vi "Set value notation.vi"(8 "error in":errorcluster, 10 "Calibration mode (disable)":u16(ring) items=["Scientific with legends", "Scientific with no legends", "Engeneering with legends", "Engeneering without legends"], 11 "VISA resource name":refnum<visa-resource-name>) -> (0 "error out":errorcluster, 3 "VISA resource name out":refnum<visa-resource-name>)   [LabVIEW 2012, in "Datron D4xxx.lvlib"]
doc: "This VI sets instrument number format."
uses:
  Datron D4xxx.lvlib
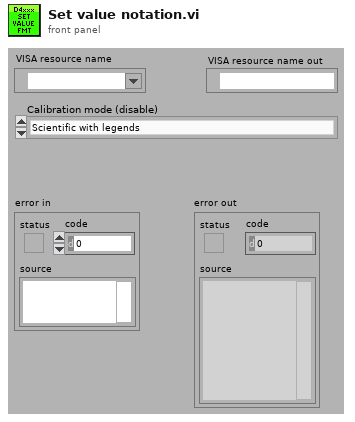
[diagram p1: front panel]
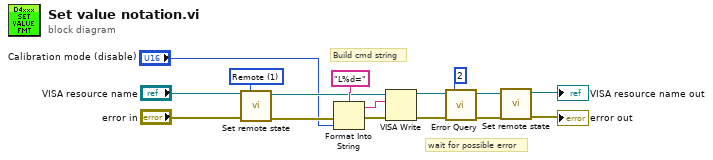
[diagram p0: block diagram]
diagram:
  w3 = u16 1 items=["Local", "Remote", "Default"] ("Remote state")
  # "Build cmd string"
  # "wait for possible error"
  n1 = call "Set remote state.vi"("error in"="error in", "Remote state"=w3, "VISA resource name"="VISA resource name") -> ("error out"=w6:errorcluster, "VISA resource name out"=w4:refnum<visa-resource-name>)  [unwired: 7 in]
  n2 = Format Into String(format string="L%d=", error in=w6, "Calibration mode (disable)") -> (resulting string=w16:string, error out=w15:errorcluster)  [unwired: 1 in]
  n3 = VISA Write(VISA resource name=w4, write buffer=w16, error in (no error)=w15) -> (VISA resource name out=w8:refnum<visa-resource-name>, error out=w9:errorcluster)  [unwired: 1 out]
  n4 = call "Error Query.vi"("error in (no error)"=w9, "Check cycles (11)"=2, "VISA resource name"=w8) -> ("error out"=w13:errorcluster, "VISA resource name out"=w11:refnum<visa-resource-name>)  [unwired: 5 in, 2 out]
  n5 = call "Set remote state.vi"("error in"=w13, "VISA resource name"=w11) -> ("error out"=→"error out":errorcluster, "VISA resource name out"=→"VISA resource name out":refnum<visa-resource-name>)  [unwired: 8 in]
